vi "pcfs_generate_UI_events.vi"(8 "error in (no error)":errorcluster, 11 "scan_panel in":refnum<class "pcfs.lvclass">) -> (0 "error out":errorcluster, 2 "update_status":refnum<event-registration>, 3 "scan_panel out":refnum<class "pcfs.lvclass">)   [LabVIEW 2015, in "pcfs.lvclass"]
uses:
  pcfs.lvclass
  pcfs_ui_events.ctl
  pcfs_ui_event_references.ctl
  pcfs.lvclass/pcfs.ctl
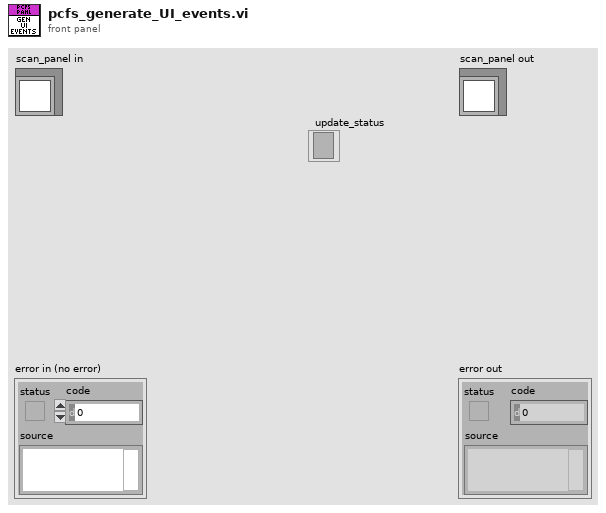
[diagram p1: front panel]
types:
  T1 = typedef "pcfs_ui_event_references.ctl" = cluster{"update_status_string_":refnum<event-registration>}
  T2 = typedef "pcfs_ui_events.ctl" = cluster{"update_scan_status":refnum<user-event>}
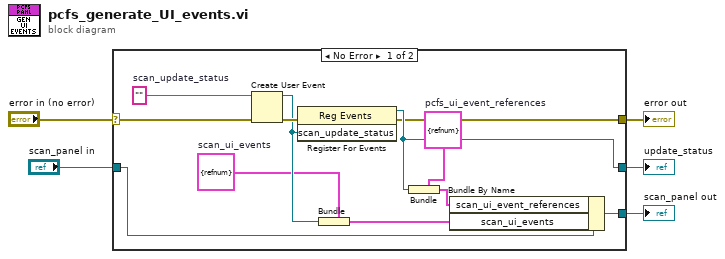
[diagram p0: block diagram]
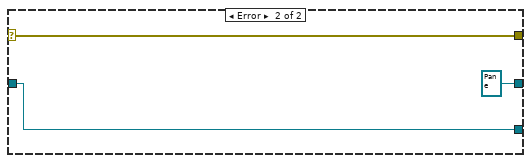
[diagram p2: hidden frame]
diagram:
  n1 = case shown="No Error" "error in (no error)" {
    selector: "error in (no error)" -> [w17 w20]
    tunnel: [w8 w20] -> w4
    tunnel: [w11 w19] -> w2
    tunnel: "scan_panel in" -> [w13 w19]
    tunnel: [w14 refnum<event-registration> refnum ("Event Registration Refnum")] -> w1
    frame No Error {
      w7 = T1 {"update_status_string_"=refnum}  # pcfs_ui_event_references
      w6 = T2 {"update_scan_status"=refnum}  # scan_ui_events
      w16 = ""  # scan_update_status
      n2 = Create User Event(user event datatype=w16, error in=w17) -> (user event=w10:refnum<user-event>, error out=w15:errorcluster)
      n3 = register-events(error in=w15, w10) -> (reference out=w14:refnum<event-registration>, error out=w8:errorcluster)  [unwired: 1 in]
      n4 = Bundle(cluster=w6, "update_scan_status"=w10) -> (w9:T2)
      n5 = Bundle(cluster=w7, "update_status_string_"=w14) -> (w12:T1)
      n6 = Bundle By Name(cluster=w13, "scan_ui_event_references"=w12, "scan_ui_events"=w9) -> (w11:refnum<class "pcfs.lvclass">)
    }
    frame Error {
    }
  }
  "error out" <- w4
  "scan_panel out" <- w2
  "update_status" <- w1
